vi "OR4x4.vi"(2 "B":bool[][](array[boolean])=[[FALSE, FALSE, FALSE, FALSE], [FALSE, FALSE, FALSE, FALSE], [FALSE, FALSE, FALSE, FALSE], [FALSE, FALSE, FALSE, FALSE]], 3 "A":bool[][](array[boolean])=[[FALSE, FALSE, FALSE, FALSE], [FALSE, FALSE, FALSE, FALSE], [FALSE, FALSE, FALSE, FALSE], [FALSE, FALSE, FALSE, FALSE]]) -> (0 "compund or":bool, 1 "z":bool[][](array[boolean]))   [LabVIEW 2012]
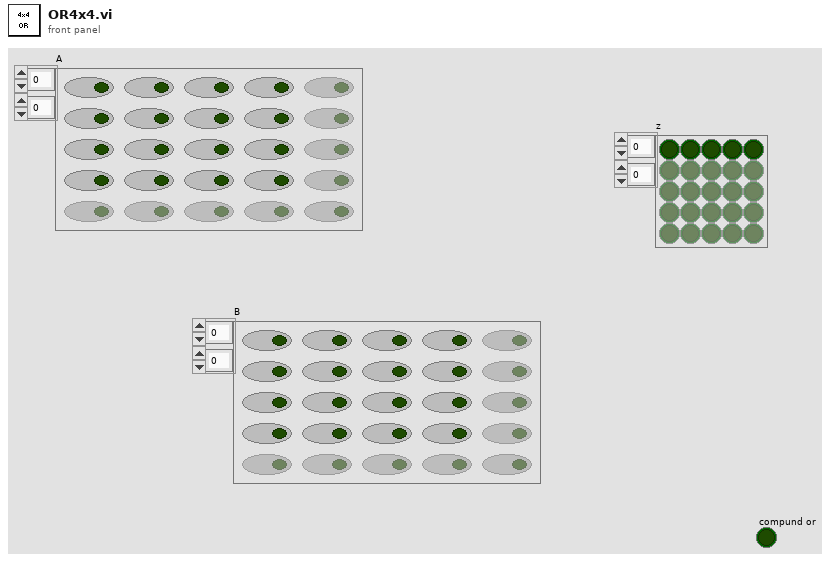
[diagram p1: front panel]
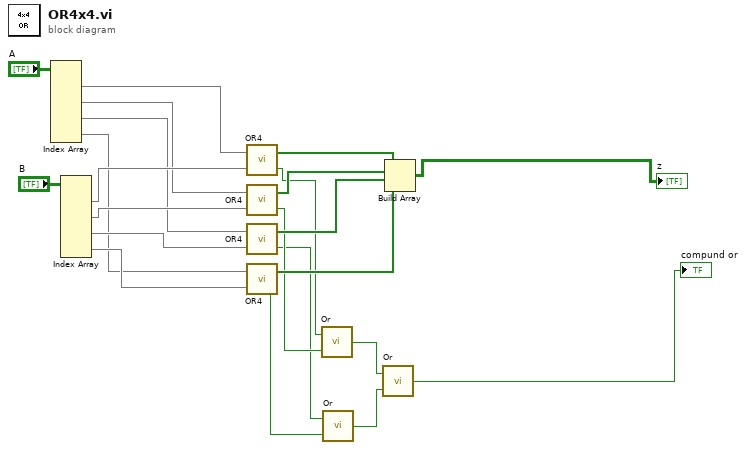
[diagram p0: block diagram]
diagram:
  n1 = Index Array(array="A") -> (element #1=w20:bool[], element #2=w3:bool[], element #3=w2:bool[], element #4=w1:bool[])  [unwired: 8 in]
  n2 = Index Array(array="B") -> (element #1=w19:bool[], element #2=w4:bool[], element #3=w18:bool[], element #4=w17:bool[])  [unwired: 8 in]
  n3 = call "OR4.vi"("B"=w19, "A"=w20) -> ("compund add"=w11:bool, "z"=w16:bool[])
  n4 = call "OR4.vi"("B"=w4, "A"=w3) -> ("compund add"=w10:bool, "z"=w15:bool[])
  n5 = call "OR4.vi"("B"=w18, "A"=w2) -> ("compund add"=w9:bool, "z"=w14:bool[])
  n6 = call "OR4.vi"("B"=w17, "A"=w1) -> ("compund add"=w8:bool, "z"=w13:bool[])
  n7 = call "Or.vi"("b"=w10, "a"=w11) -> ("x"=w6:bool)
  n8 = call "Or.vi"("b"=w8, "a"=w9) -> ("x"=w7:bool)
  n9 = call "Or.vi"("b"=w7, "a"=w6) -> ("x"=→"compund or":bool)
  n10 = Build Array(w16, w15, w14, w13) -> (→"z":bool[][])
